vi "controlMotionControlThreshold.vi"(7 "Set":bool, 8 "error in":errorcluster, 9 "threshold":i32, 10 "axis in":u8, 11 "connection ID":refnum<k5>) -> (0 "error out":errorcluster, 1 "threshold out":i32, 2 "axis out":u8, 3 "connection ID":refnum<k5>)   [LabVIEW 2016]
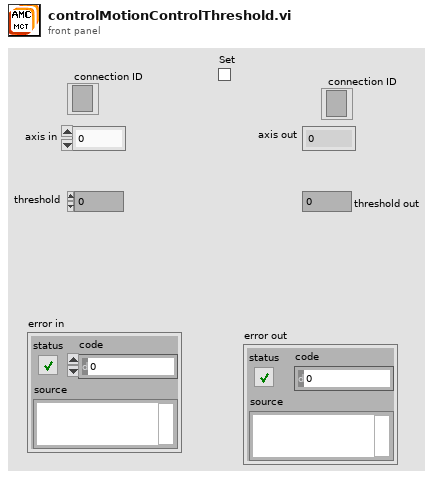
[diagram p1: front panel]
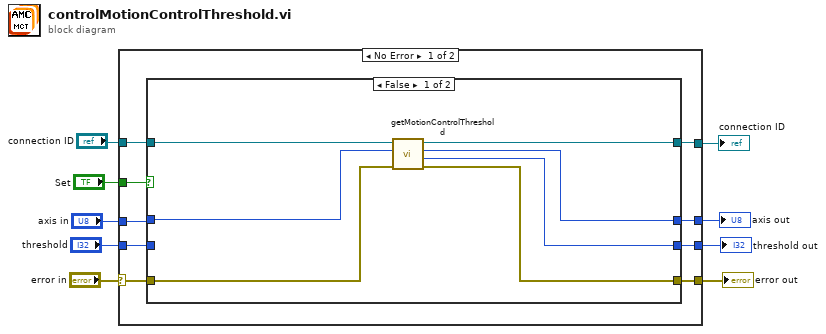
[diagram p0: block diagram]
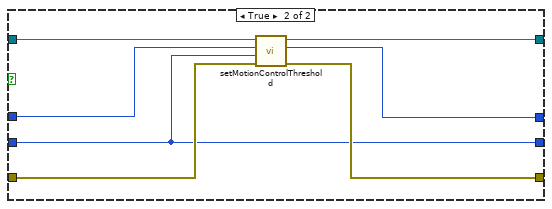
[diagram p2: hidden frame]
diagram:
  n1 = case shown="No Error" "error in" {
    selector: "error in" -> [w12 w36]
    tunnel: "axis in" -> [w16 w35]
    tunnel: [w13 w36] -> w8
    tunnel: [w14 w35] -> w7
    tunnel: "Set" -> [w17 _]
    tunnel: [w15 w34] -> w5
    tunnel: "connection ID" -> [w18 w34]
    tunnel: "threshold" -> [w11 w33]
    tunnel: [w10 w33] -> w1
    frame No Error {
      n2 = case shown="False" w17 {
        tunnel: [w24 w31] -> w15
        tunnel: w18 -> [w25 w32]
        tunnel: w16 -> [w23 w28]
        tunnel: [w22 w27] -> w14
        tunnel: [w20 w30] -> w13
        tunnel: w12 -> [w21 w29]
        tunnel: w11 -> [_ w26]
        tunnel: [w19 w26] -> w10
        frame False {
          n3 = call "getMotionControlThreshold.vi"("error in"=w21, "axis"=w23, "connection ID"=w25) -> ("error out"=w20:errorcluster, "range"=w19:i32, "axis_out"=w22:i32, "connection ID"=w24:refnum<k5>)  [unwired: 5 in]
        }
        frame True {
          n4 = call "setMotionControlThreshold.vi"("error in"=w29, "threshold"=w26, "axis"=w28, "connection ID"=w32) -> ("error out"=w30:errorcluster, "axis_out"=w27:i32, "connection ID"=w31:refnum<k5>)  [unwired: 5 in]
        }
      }
    }
    frame Error {
    }
  }
  "error out" <- w8
  "axis out" <- w7
  "connection ID" <- w5
  "threshold out" <- w1
